vi "Handle Response.vi"(7 "Processing In":refnum<class "Processing.lvclass">, 11 "GodotHeaders in":refnum<class "GodotHeaders.lvclass">) -> (0 "error out":errorcluster, 5 "Processing":refnum<class "Processing.lvclass">)   [LabVIEW 2020, in "FormulaG.lvlib" / "GodotHeaders.lvclass"]
uses:
  GodotHeaders.lvclass
  <vilib>/IlluminatedG/IG HTTP Server/HTTP Server/Processing/Processing.lvclass
  <vilib>/IlluminatedG/IG HTTP Server/HTTP Server/Processing/Processing.lvclass/Processing.ctl
  <vilib>/IlluminatedG/IG HTTP Utils/HTTP Utils/Response/Response.lvclass
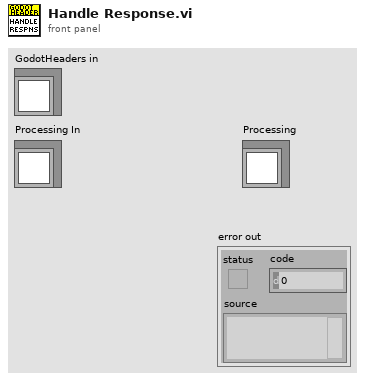
[diagram p1: front panel]
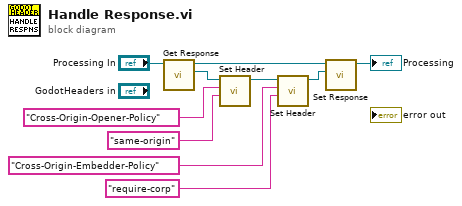
[diagram p0: block diagram]
diagram:
  n1 = call <vilib>:"Get Response.vi"("Processing in"="Processing In") -> ("Response"=w10:refnum<class "Response.lvclass">, "Processing out"=w4:refnum<class "Processing.lvclass">)  [unwired: 9 in]
  n2 = call <vilib>:"Set Header.vi"("Value"="same-origin" ("Header"), "Header"="Cross-Origin-Opener-Policy", "Response in"=w10) -> ("Response out"=w7:refnum<class "Response.lvclass">)  [unwired: 6 in, 2 out]
  n3 = call <vilib>:"Set Header.vi"("Value"="require-corp" ("Header"), "Header"="Cross-Origin-Embedder-Policy", "Response in"=w7) -> ("Response out"=w3:refnum<class "Response.lvclass">)  [unwired: 6 in, 2 out]
  n4 = call <vilib>:"Set Response.vi"("Response"=w3, "Processing in"=w4) -> ("Processing out"=→"Processing":refnum<class "Processing.lvclass">)  [unwired: 9 in]
